vi "Logger.vi"(8 "error in (no error)":errorcluster) -> (0 "error out":errorcluster)   [LabVIEW 2021]
uses:
  QueueEnum.ctl
  ToViewQueueData.ctl
  ViewUpdateEnum.ctl
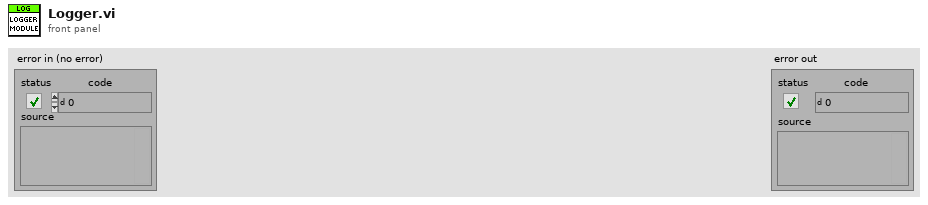
[diagram p1: front panel]
types:
  T1 = enum32{"Invalid", "Standard", "Closed", "Hidden", "Minimized", "Maximized"}
  T2 = enum16{"open", "replace", "create", "open or create", "replace or create", "replace or create with confirmation"}
  T3 = typedef "ViewUpdateEnum.ctl" = enum16{"Init", "OneButtonMessage", "Exit", "UpdateButtonsEnabled", "UpdateGraph", "UpdateConnectionStatus"}
  T4 = typedef "ToViewQueueData.ctl" = cluster{"DataToUpdate":T3, "ConnectionStatus":bool, "GraphData":dbl[][], "Message":string}
  T5 = typedef "QueueEnum.ctl" = enum16{"Obtain Queue", "Get Queue Ref", "Flush Queue", "Release Queue"}
  T6 = typedef "ToLoggerQueueCluster.ctl" = cluster{"Command":T7, "Data":dbl[][], "Path":path}
  T7 = typedef "LoggerEnum.ctl" = enum16{"StartLogging", "StopLogging", "ReadData", "SendData", "WriteData", "Exit"}
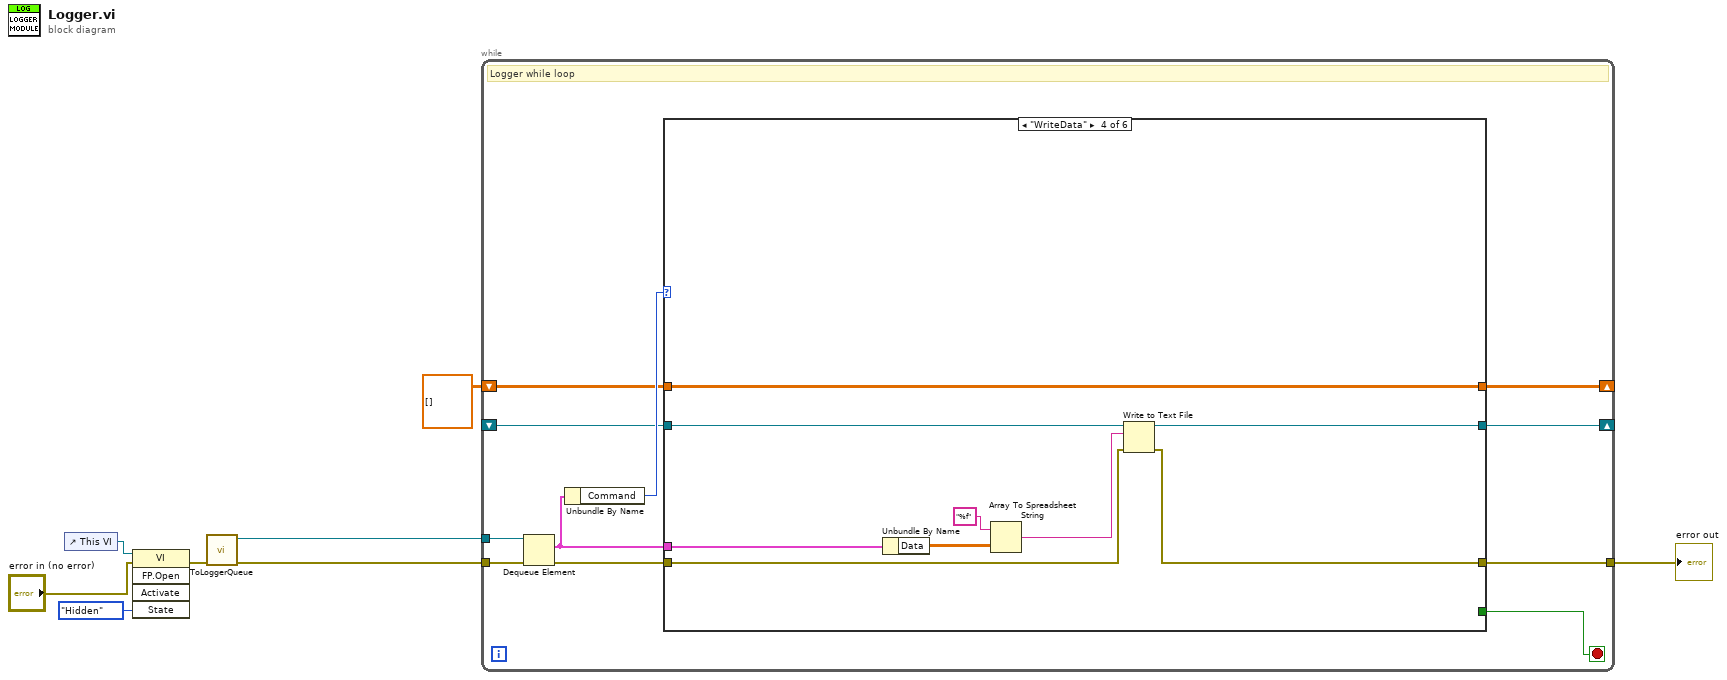
[diagram p0: block diagram]
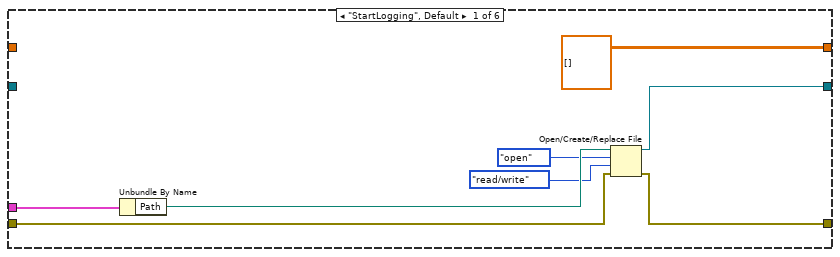
[diagram p2: hidden frame]
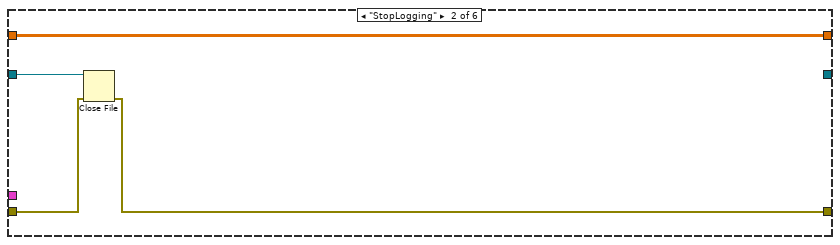
[diagram p3: hidden frame]
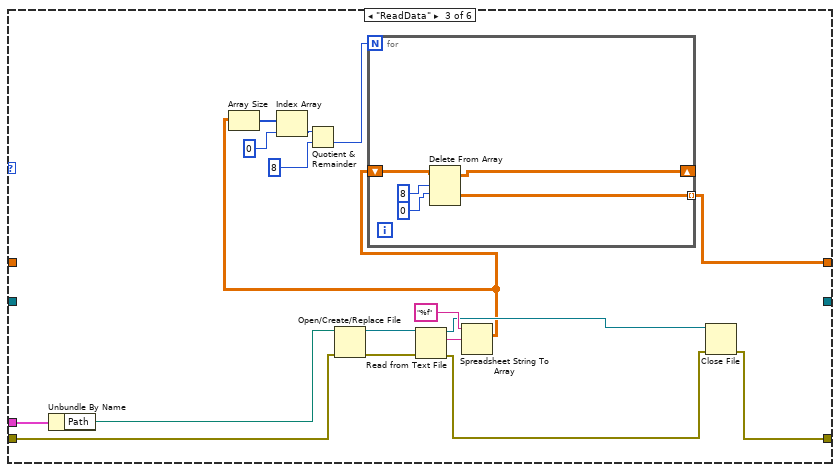
[diagram p4: hidden frame]
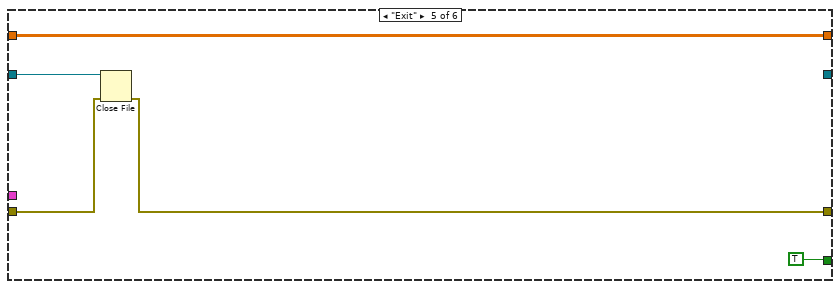
[diagram p5: hidden frame]
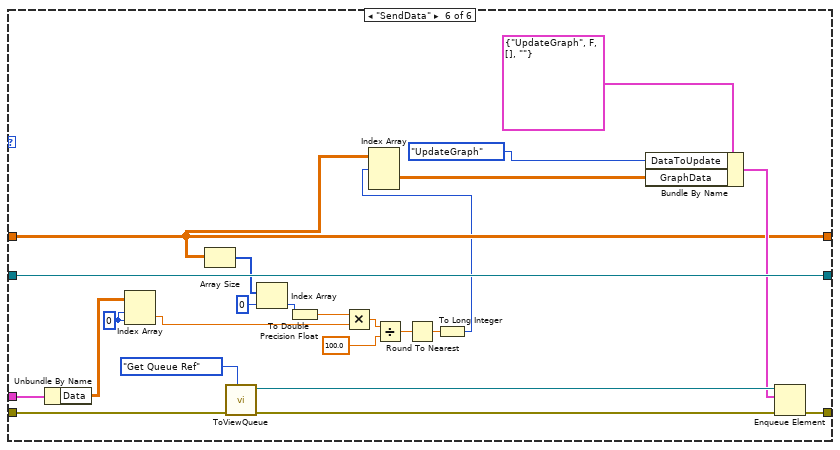
[diagram p6: hidden frame]
diagram:
  n1 = control-ref of="This VI"() -> (w8:refnum<vi>)
  n2 = invoke class="VI" method="FP.Open"(reference=w8, error in="error in (no error)", "State"=T1."Hidden") -> (error out=w4:errorcluster)  [unwired: 2 in, 4 out]
  n3 = call "ToLoggerQueue.vi"("error in (no error)"=w4) -> ("error out"=w2:errorcluster, "queue out"=w3:refnum<queue>)  [unwired: 9 in]
  n4 = while {
    tunnel: w2 -> [w17]
    tunnel: [w19] -> w5
    tunnel: w3 -> [w15]
    shift-right: [w12] -> _
    shift-left: _ -> [w11]
    shift-right: [w10] -> _
    shift-left: dbl[][][] [] -> [w9]
    stop <- w18 stop-if-true
    # "Logger while loop"
    n5 = Dequeue Element(queue=w15, error in (no error)=w17) -> (element=w13:T6, error out=w16:errorcluster)  [unwired: 1 in, 2 out]
    n6 = Unbundle By Name(w13) -> ("Command"=w14:T7)
    n7 = case shown="\"WriteData\"" w14 {
      tunnel: w16 -> [w23 w30 w46 w59 w65 w87]
      tunnel: [w21 w29 w40 w58 w64 w83] -> w19
      tunnel: [_ _ _ _ TRUE _] -> w18
      tunnel: w13 -> [w27 _ w43 w61 _ w81]
      tunnel: [w22 _ _ w60 _ w91] -> w12
      tunnel: w11 -> [_ w31 _ w62 w66 w91]
      tunnel: [dbl[][][] [] w28 w38 w55 w63 w78] -> w10
      tunnel: w9 -> [_ w28 _ w55 w63 w78]
      frame "StartLogging", Default {
        n8 = Unbundle By Name(w27) -> ("Path"=w26:path)
        n9 = Open/Create/Replace File(file path (use dialog)=w26, error in=w23, operation (0:open)=T2."open", access (0:read/write)=enum16{"read/write", "read-only", "write-only"}."read/write") -> (refnum out=w22:refnum<file>, error out=w21:errorcluster)  [unwired: 2 in, 1 out]
      }
      frame "StopLogging" {
        n10 = Close File(refnum=w31, error in=w30) -> (error out=w29:errorcluster)  [unwired: 1 out]
      }
      frame "ReadData" {
        n11 = Unbundle By Name(w43) -> ("Path"=w42:path)
        n12 = Open/Create/Replace File(file path (use dialog)=w42, error in=w46) -> (refnum out=w44:refnum<file>, error out=w45:errorcluster)  [unwired: 4 in, 1 out]
        n13 = Read from Text File(file (use dialog)=w44, error in=w45) -> (refnum out=w39:refnum<file>, text=w47:string, error out=w41:errorcluster)  [unwired: 2 in, 1 out]
        n14 = Spreadsheet String To Array(format string="%f", spreadsheet string=w47) -> (array=w37:dbl[][])  [unwired: 2 in]
        n15 = Array Size(array=w37) -> (size(s)=w36:i32[])
        n16 = Index Array(array=w36, index=0) -> (element=w34:i32)
        n17 = Quotient & Remainder(x=w34, y=8) -> (floor(x/y)=w32:i32)  [unwired: 1 out]
        n18 = for {
          N: w32 -> [_]
          shift-right: [w52] -> _
          shift-left: w37 -> [w53]
          tunnel: [w51] -> w38 mode=indexing
          n19 = Delete From Array(array=w53, length=8, index (row)=0) -> (deleted portion=w51:dbl[][], array with subset deleted=w52:dbl[][])  [unwired: 1 in]
        }
        n20 = Close File(refnum=w39, error in=w41) -> (error out=w40:errorcluster)  [unwired: 1 out]
      }
      frame "WriteData" {
        n21 = Unbundle By Name(w61) -> ("Data"=w57:dbl[][])
        n22 = Array To Spreadsheet String(array=w57, 3:"%f" ("format string")) -> (spreadsheet string=w54:string)  [unwired: 1 in]
        n23 = Write to Text File(file (use dialog)=w62, text=w54, error in=w59) -> (refnum out=w60:refnum<file>, error out=w58:errorcluster)  [unwired: 1 in, 1 out]
      }
      frame "Exit" {
        n24 = Close File(refnum=w66, error in=w65) -> (error out=w64:errorcluster)  [unwired: 1 out]
      }
      frame "SendData" {
        w79 = 0 ("index")
        n25 = Unbundle By Name(w81) -> ("Data"=w80:dbl[][])
        n26 = Index Array(array=w80, index (row)=w79, index (col)=w79) -> (element=w74:dbl)
        n27 = Array Size(array=w78) -> (size(s)=w76:i32[])
        n28 = call "ToViewQueue.vi"("Enum"=QueueEnum."Get Queue Ref", "error in (no error)"=w87) -> ("error out"=w90:errorcluster, "queue out"=w89:refnum<queue>)  [unwired: 8 in]
        n29 = Index Array(array=w76, index=0) -> (element=w75:i32)
        n30 = To Double Precision Float(number=w75) -> (double precision float=w73:dbl)
        n31 = Multiply(x=w73, y=w74) -> (x*y=w72:dbl)
        n32 = Divide(x=w72, y=100.0) -> (x/y=w70:dbl)
        n33 = Round To Nearest(number=w70) -> (nearest integer value=w69:dbl)
        n34 = To Long Integer(number=w69) -> (32bit integer=w68:i32)
        n35 = Index Array(array=w78, index (dim 0)=w68) -> (element=w82:dbl[][])  [unwired: 2 in]
        n36 = Bundle By Name(cluster=T4 {"DataToUpdate"=enum."UpdateGraph", "ConnectionStatus"=FALSE, "GraphData"=[], "Message"=""} ("element"), "DataToUpdate"=ViewUpdateEnum."UpdateGraph", "GraphData"=w82) -> (w86:T4)
        n37 = Enqueue Element(queue=w89, element=w86, error in (no error)=w90) -> (error out=w83:errorcluster)  [unwired: 1 in, 2 out]
      }
    }
  }
  "error out" <- w5
